vi "byte array to int(1).vi"(1 "unsigned byte array":u8[](array[numeric]), 2 "索引":i32) -> (0 "数值":i16)   [LabVIEW 2018]
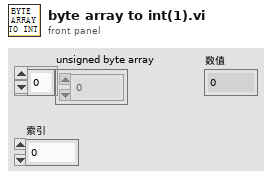
[diagram p1: front panel]
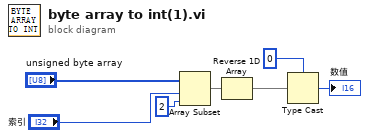
[diagram p0: block diagram]
diagram:
  n1 = Array Subset(array="unsigned byte array", index="索引", length=2 ("长度")) -> (w6:u8[])
  n2 = Reverse 1D Array(array=w6) -> (reversed array=w7:u8[])
  n3 = Type Cast(type=i16 0, x=w7) -> (*(type *) &x=→"数值":i16)
